vi "Stop Core.vi"(10 "final error code":i32, 11 "CS++GoBangClient in":refnum<class "CS++GoBangClient.lvclass">) -> (3 "CS++GoBangClient out":refnum<class "CS++GoBangClient.lvclass">)   [LabVIEW 2013, in "GoBang.lvlib" / "CS++GoBangClient.lvclass"]
doc: "(<B>Filename</B>: Actor Framework.lvlib:Actor.lvclass:Stop Core.vi)\n\nDefines what the actor does before it stops. Use the <B>final error code</B> input to determine whether the actor shut down in response to an error.\n\nBy default, this method does nothing. A descendant class may override it to define behavior, such as shutting down any processes the actor initiated in its override of the Actor Core method."
uses:
  CS++GoBangClient.lvclass
  Core/Actors/CS++BaseActor/CS++BaseActor.lvclass
  CS++GoBangClient.lvclass/CS++GoBangClient.ctl
  <vilib>/ActorFramework/Message Enqueuer/Message Enqueuer.lvclass/Message Enqueuer.ctl
  Core/Classes/CS++ProcessVariables/PVConnection/PVConnection.lvclass
  <vilib>/ActorFramework/Message Enqueuer/Enqueue.vi
  <vilib>/ActorFramework/Message Priority Queue/Priority Enqueue.vi
  <vilib>/ActorFramework/Stop Msg/Stop Msg.lvclass
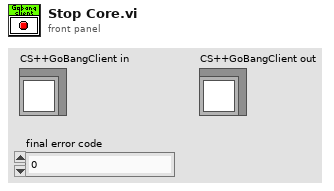
[diagram p1: front panel]
types:
  T1 = cluster{"JoinGame":refnum<class "PVConnection.lvclass">, "UpdateBoard":refnum<class "PVConnection.lvclass">}
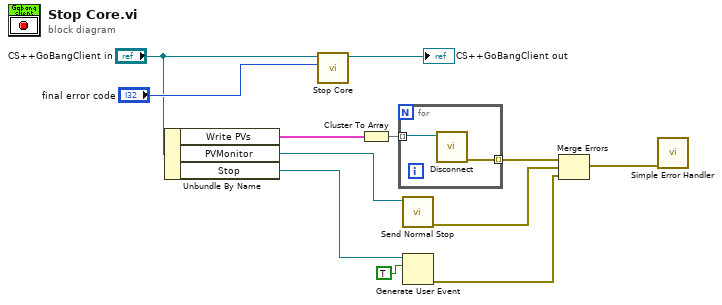
[diagram p0: block diagram]
diagram:
  n1 = Unbundle By Name("CS++GoBangClient in") -> ("Write PVs"=w9:T1, "PVMonitor"=w7:refnum<class "Message Enqueuer.lvclass">, "Stop"=w3:refnum<user-event>)
  n2 = call-parent "Stop Core.vi"("final error code"="final error code", "CS++BaseActor in"="CS++GoBangClient in") -> ("CS++BaseActor out"=→"CS++GoBangClient out":refnum<class "CS++GoBangClient.lvclass">)  [unwired: 9 in]
  n3 = Cluster To Array(cluster=w9) -> (array=w8:refnum<class "PVConnection.lvclass">[])
  n4 = for {
    tunnel: w8 -> [w14] mode=indexing
    tunnel: [w13] -> w6 mode=indexing
    n5 = call-dynamic "Disconnect.vi"("PVConnection in"=w14) -> ("error out"=w13:errorcluster)  [unwired: 9 in, 1 out]
  }
  n6 = call <vilib>:"Send Normal Stop.vi"("Message Enqueuer"=w7) -> ("error out"=w5:errorcluster)  [unwired: 10 in]
  n7 = Generate User Event(user event=w3, event data cluster=TRUE ("event data")) -> (error out=w1:errorcluster)  [unwired: 2 in, 1 out]
  n8 = Merge Errors(w6, w5, w1) -> (w4:errorcluster)
  n9 = call <vilib>:"Simple Error Handler.vi"("error in (no error)"=w4) -> ()  [unwired: 4 in, 5 out]
